vi "Func-Math-Finder-18032016.vi"(4 "All Fn-Math":string[](array[string]), 6 "All Fn Name":string[](array[string]), 7 "Func Name":string, 8 "error in (no error)":errorcluster, 9 "Functions Definition":string[][](table), 11 "Get Tagged String":string) -> (0 "error out":errorcluster, 1 "is empty?":string, 2 "Expression":string)   [LabVIEW 2014]
doc: "This VI takes tagged string from SBML parser.vi as input and translate it into kinetic law. It supports the following five mathematical functions:\n+, -, *, /, pow\n\nDesigned by HB\nhaba@dtu.dk"
uses:
  <vilib>/regexp/Match Regular Expression.xnode
panel:
  out "Fn Variables":string[](array[string])
  out "Nest Fn?":string
  out "Current Args":string[](array[string])
  out "RHS ex":string
  out "Inter. exp":string
  in  "RHS":string
  in  "LHS":string
  # "multiplySOP1k1, addSOP2S1, S2EOP2, subSOP2k1, 4EOP2EOP1"
  # "SOP1 + x 2 EOP1"
  # "SOP1 + SOP2 * a b EOP2 c EOP1"
  # "SOP1 + c SOP2 * a b EOP2 EOP1"
  # "SOP1 + SOP2 * a SOP3 pow x 2 EOP3 EOP2 SOP2 * b x EOP2 c EOP1"
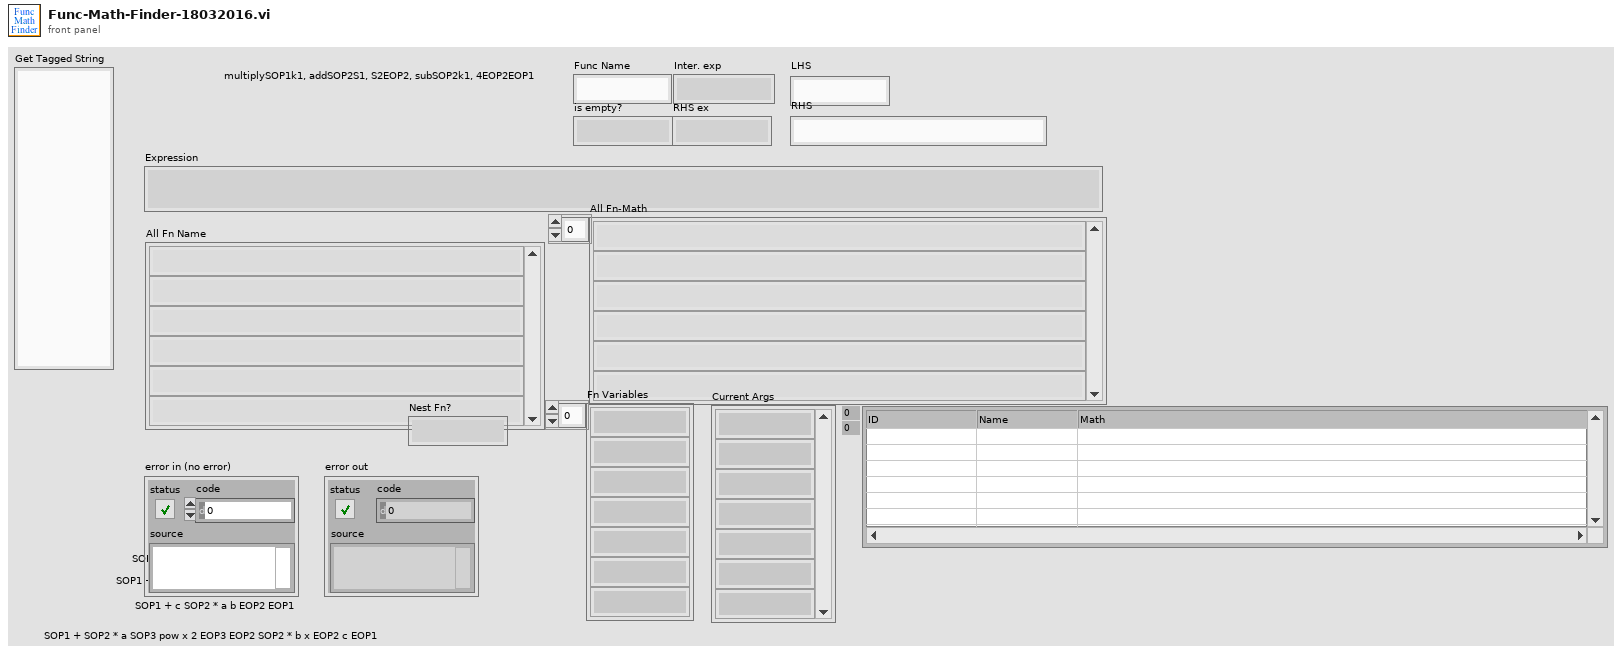
[diagram p1: front panel]
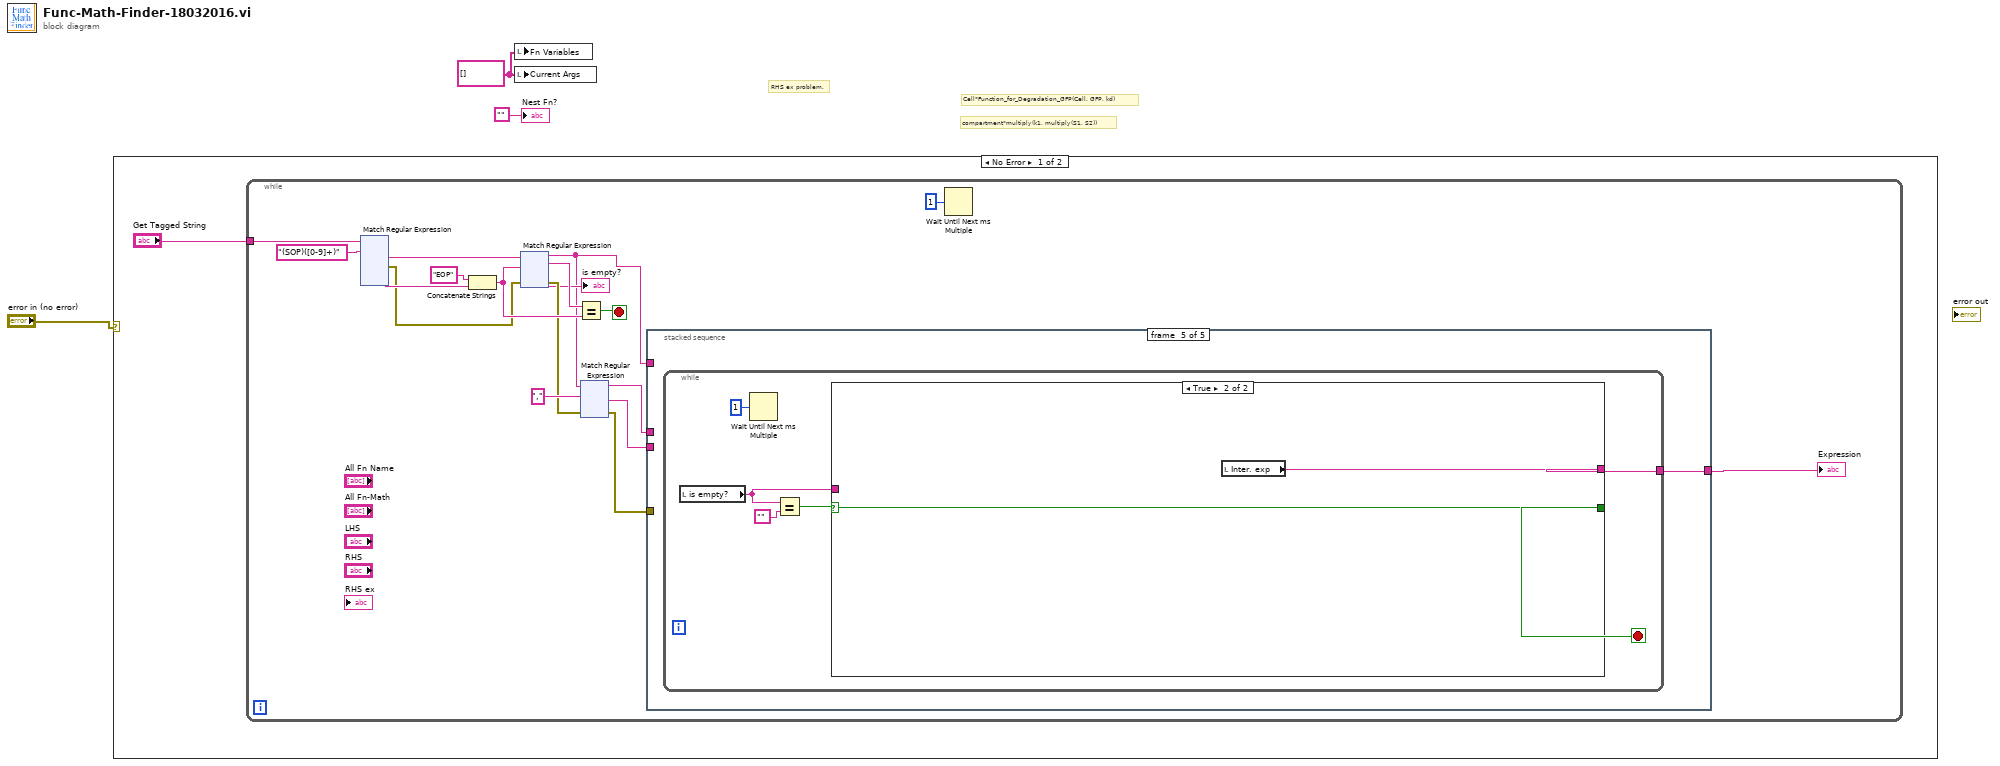
[diagram p0: block diagram]
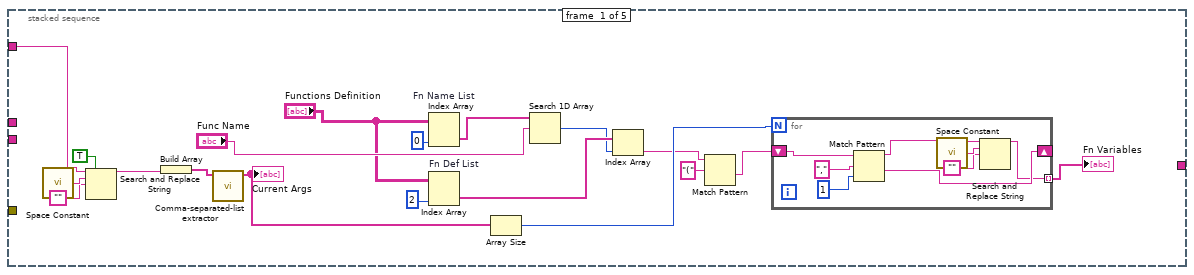
[diagram p2: hidden frame]
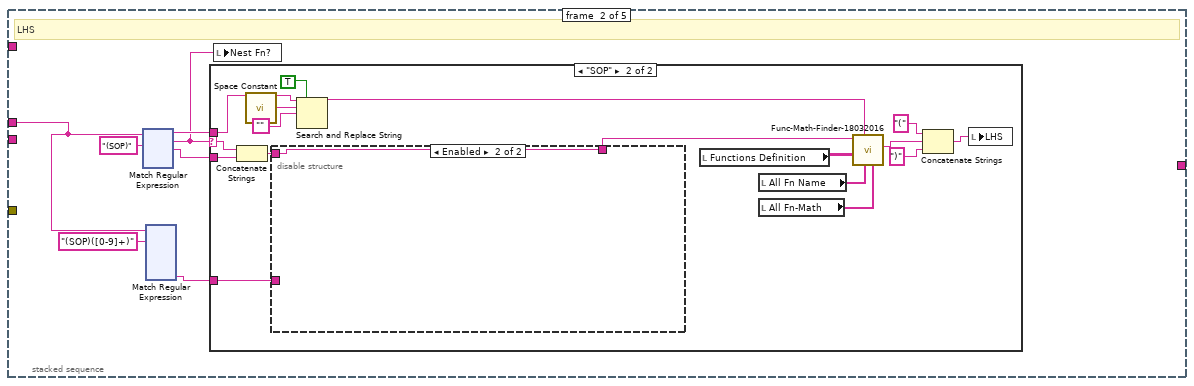
[diagram p3: hidden frame]
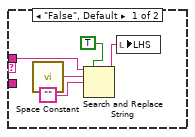
[diagram p4: hidden frame]
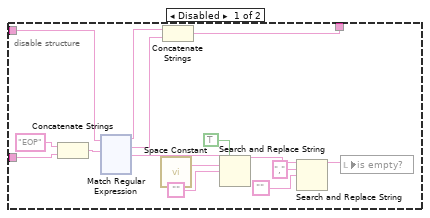
[diagram p5: hidden frame]
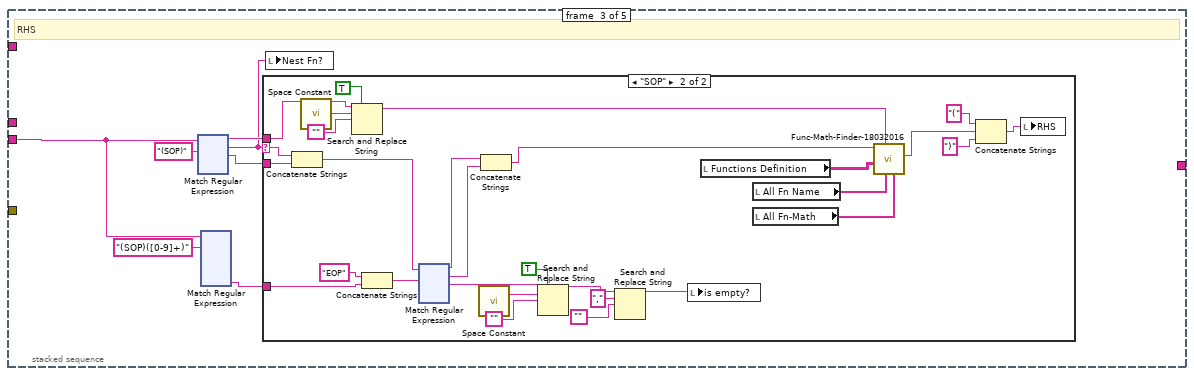
[diagram p6: hidden frame]
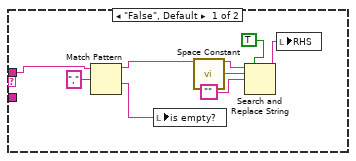
[diagram p7: hidden frame]
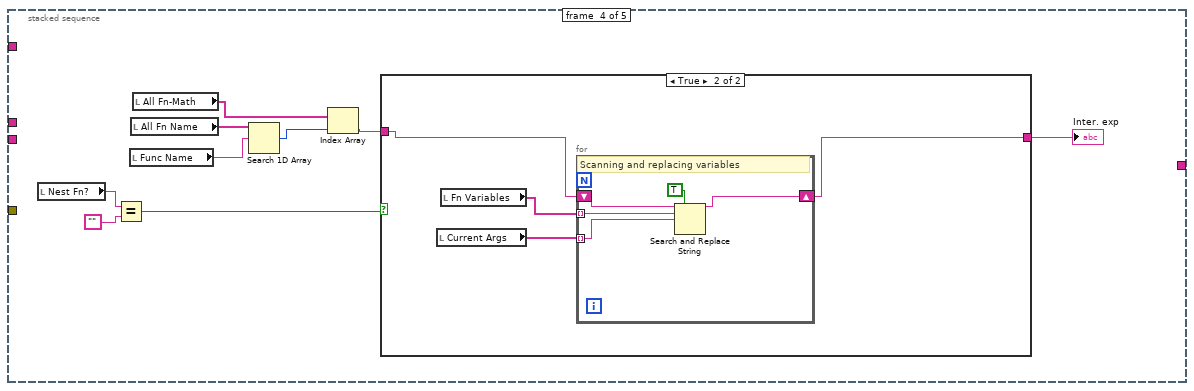
[diagram p8: hidden frame]
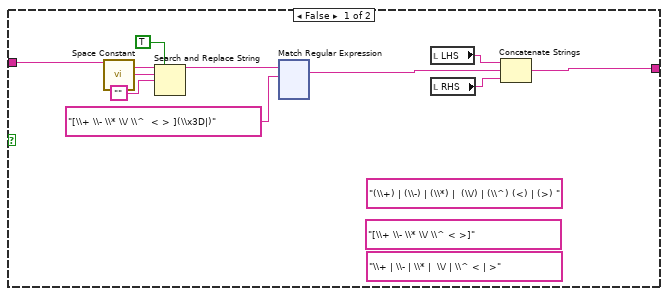
[diagram p9: hidden frame]
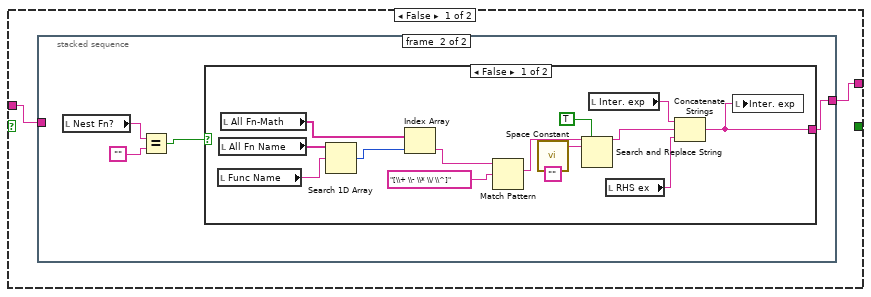
[diagram p10: hidden frame]
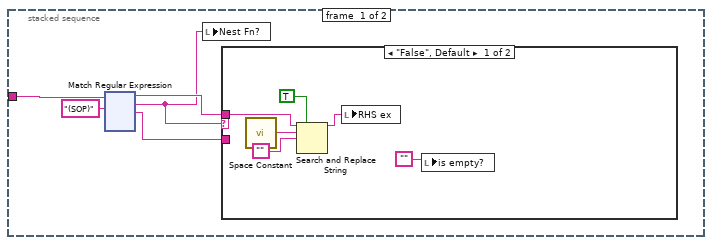
[diagram p11: hidden frame]
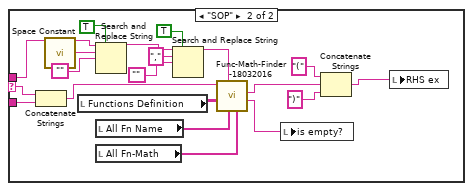
[diagram p12: hidden frame]
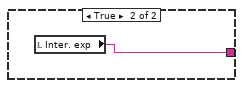
[diagram p13: hidden frame]
diagram:
  w1 = string[] [] ("Current Args")
  # "compartment*multiply(k1, multiply(S1, S2))"
  # "Cell*Function_for_Degradation_GFP(Cell, GFP, kd)"
  # "RHS ex problem."
  n1 = case shown="No Error" "error in (no error)" {
    frame No Error {
      n2 = while {
        tunnel: "Get Tagged String" -> [w14]
        stop <- w20 stop-if-true
        n3 = xnode "Match Regular Expression"("input string"=w14, "regular expression"="(SOP)([0-9]+)") -> ("after match"=w17:string, "error out"=w13:errorcluster, "submatch 2"=w16:string)  [unwired: 4 in, 4 out]
        n4 = Concatenate Strings("EOP" ("regular expression"), w16) -> (w21:string)
        n5 = xnode "Match Regular Expression"("input string"=w17, "regular expression"=w21, "error in"=w13) -> ("before match"=w6:string, "whole match"=w19:string, "after match"=→"is empty?":string, "error out"=w12:errorcluster)  [unwired: 3 in, 1 out]
        n6 = Equal?(x=w19, y=w21) -> (x = y?=w20:bool)
        n7 = xnode "Match Regular Expression"("input string"=w6, "regular expression"="," ("Oprts Lst"), "error in"=w12) -> ("before match"=w11:string, "after match"=w9:string, "error out"=w10:errorcluster)  [unwired: 3 in, 2 out]
        n8 = stacked-sequence {
          tunnel: w11 -> [_ w51 _ _ _]
          tunnel: w10 -> [_ _ _ _ _]
          tunnel: w9 -> [_ _ w442 _ _]
          tunnel: [_ _ _ _ w971] -> w8
          tunnel: w6 -> [w23 _ _ _ _]
          frame #0 {
            n9 = call <vilib>:"Space Constant.vi"() -> ("String"=w26:string)
            n10 = Search and Replace String(replace all?=TRUE ("replace all? (F)"), input string=w23, search string=w26, replace string="") -> (result string=w28:string)  [unwired: 4 in, 3 out]
            n11 = Build Array(w28) -> (w24:string[])
            n12 = call "Comma-separated-list extractor.vi"("In_list"=w24) -> ("List_Out"=w39:string[])  [unwired: 6 in, 1 out]
            "Current Args" <- w39
            n13 = Index Array "Fn Name List"(array="Functions Definition", index (col)=0 ("disabled index (col)")) -> (element=w29:string[])  [unwired: 1 in]
            n14 = Index Array "Fn Def List"(array="Functions Definition", index (col)=2 ("disabled index (col)")) -> (element=w34:string[])  [unwired: 1 in]
            n15 = Array Size(array=w39) -> (size(s)=w40:i32)
            n16 = Search 1D Array(1D array=w29, element="Func Name") -> (index of element=w33:i32)  [unwired: 1 in]
            n17 = Index Array(array=w34, index=w33) -> (element=w38:string)
            n18 = Match Pattern(string=w38, regular expression="(") -> (after substring=w36:string)  [unwired: 1 in, 3 out]
            n19 = for {
              N: w40 -> [_]
              shift-right: [w46] -> _
              shift-left: w36 -> [w49]
              tunnel: [w42] -> w35 mode=indexing
              n20 = Match Pattern(string=w49, regular expression="," ("search string/char (-)"), offset (0)=1) -> (before substring=w43:string, after substring=w46:string)  [unwired: 2 out]
              n21 = call <vilib>:"Space Constant.vi"() -> ("String"=w45:string)
              n22 = Search and Replace String(input string=w43, search string=w45, replace string="") -> (result string=w42:string)  [unwired: 5 in, 3 out]
            }
            "Fn Variables" <- w35
          }
          frame #1 {
            # "LHS"
            n23 = xnode "Match Regular Expression"("input string"=w51, "regular expression"="(SOP)") -> ("before match"=w54:string, "whole match"=w50:string, "after match"=w55:string)  [unwired: 4 in, 2 out]
            n24 = xnode "Match Regular Expression"("input string"=w51, "regular expression"="(SOP)([0-9]+)") -> ("submatch 2"=w52:string)  [unwired: 4 in, 6 out]
            n25 = case shown="\"SOP\"" w50 {
              selector: w50 -> [_ w195]
              tunnel: w54 -> [w175 w186]
              tunnel: w55 -> [_ w194]
              tunnel: w52 -> [_ w182]
              frame "False", Default {
                n26 = call <vilib>:"Space Constant.vi"() -> ("String"=w177:string)
                n27 = Search and Replace String(replace all?=TRUE ("replace all? (F)"), input string=w175, search string=w177, replace string="" ("string")) -> (result string=w174:string)  [unwired: 4 in, 3 out]
                n28 = local write "LHS"(w174) -> ()
              }
              frame "SOP" {
                n29 = Concatenate Strings(w195, w194) -> (w181:string)
                n30 = call <vilib>:"Space Constant.vi"() -> ("String"=w187:string)
                n31 = disable-structure shown="Enabled" {
                  disable-tunnel: w182 -> [w209 _]
                  disable-tunnel: w181 -> [w199 w325]
                  disable-tunnel: [w198 w325] -> w180
                  frame Disabled {
                    n32 = Concatenate Strings("EOP" ("regular expression"), w209) -> (w208:string)
                    n33 = xnode "Match Regular Expression"("input string"=w199, "regular expression"=w208) -> ("before match"=w200:string, "whole match"=w201:string, "after match"=w203:string)  [unwired: 4 in, 2 out]
                    n34 = call <vilib>:"Space Constant.vi"() -> ("String"=w206:string)
                    n35 = Concatenate Strings(w200, w201) -> (w198:string)
                    n36 = Search and Replace String(replace all?=TRUE ("replace all? (F)"), input string=w203, search string=w206, replace string="" ("string")) -> (result string=w205:string)  [unwired: 4 in, 3 out]
                    n37 = Search and Replace String(input string=w205, search string=",", replace string="" ("string")) -> (result string=w202:string)  [unwired: 5 in, 3 out]
                    n38 = local write "is empty?"(w202) -> ()
                  }
                  frame Enabled {
                  }
                }
                n39 = Search and Replace String(replace all?=TRUE ("replace all? (F)"), input string=w186, search string=w187, replace string="" ("string")) -> (result string=w185:string)  [unwired: 4 in, 3 out]
                n40 = local read "Functions Definition"() -> (w179:string[][])
                n41 = local read "All Fn Name"() -> (w184:string[])
                n42 = local read "All Fn-Math"() -> (w183:string[])
                n43 = call "Func-Math-Finder-18032016.vi"("All Fn-Math"=w183, "All Fn Name"=w184, "Func Name"=w185, "Functions Definition"=w179, "Get Tagged String"=w180) -> ("Expression"=w190:string)  [unwired: 4 in, 2 out]
                n44 = Concatenate Strings("(" ("string"), w190, ")" ("string")) -> (w191:string)
                n45 = local write "LHS"(w191) -> ()
              }
            }
            n46 = local write "Nest Fn?"(w50) -> ()
          }
          frame #2 {
            # "RHS"
            n47 = xnode "Match Regular Expression"("input string"=w442, "regular expression"="(SOP)") -> ("before match"=w444:string, "whole match"=w440:string, "after match"=w445:string)  [unwired: 4 in, 2 out]
            n48 = xnode "Match Regular Expression"("input string"=w442, "regular expression"="(SOP)([0-9]+)") -> ("submatch 2"=w441:string)  [unwired: 4 in, 6 out]
            n49 = case shown="\"SOP\"" w440 {
              selector: w440 -> [_ w600]
              tunnel: w444 -> [w567 w591]
              tunnel: w445 -> [_ w599]
              tunnel: w441 -> [_ w586]
              frame "False", Default {
                n50 = Match Pattern(string=w567, regular expression=",") -> (before substring=w565:string, after substring=w564:string)  [unwired: 1 in, 2 out]
                n51 = local write "is empty?"(w564) -> ()
                n52 = call <vilib>:"Space Constant.vi"() -> ("String"=w570:string)
                n53 = Search and Replace String(replace all?=TRUE ("replace all? (F)"), input string=w565, search string=w570, replace string="" ("string")) -> (result string=w568:string)  [unwired: 4 in, 3 out]
                n54 = local write "RHS"(w568) -> ()
              }
              frame "SOP" {
                n55 = Concatenate Strings(w600, w599) -> (w576:string)
                n56 = call <vilib>:"Space Constant.vi"() -> ("String"=w592:string)
                n57 = Search and Replace String(replace all?=TRUE ("replace all? (F)"), input string=w591, search string=w592, replace string="" ("string")) -> (result string=w590:string)  [unwired: 4 in, 3 out]
                n58 = Concatenate Strings("EOP" ("regular expression"), w586) -> (w585:string)
                n59 = xnode "Match Regular Expression"("input string"=w576, "regular expression"=w585) -> ("before match"=w577:string, "whole match"=w578:string, "after match"=w580:string)  [unwired: 4 in, 2 out]
                n60 = call <vilib>:"Space Constant.vi"() -> ("String"=w583:string)
                n61 = Concatenate Strings(w577, w578) -> (w575:string)
                n62 = Search and Replace String(replace all?=TRUE ("replace all? (F)"), input string=w580, search string=w583, replace string="" ("string")) -> (result string=w582:string)  [unwired: 4 in, 3 out]
                n63 = Search and Replace String(input string=w582, search string=",", replace string="" ("string")) -> (result string=w579:string)  [unwired: 5 in, 3 out]
                n64 = local write "is empty?"(w579) -> ()
                n65 = local read "Functions Definition"() -> (w572:string[][])
                n66 = local read "All Fn Name"() -> (w589:string[])
                n67 = local read "All Fn-Math"() -> (w588:string[])
                n68 = call "Func-Math-Finder-18032016.vi"("All Fn-Math"=w588, "All Fn Name"=w589, "Func Name"=w590, "Functions Definition"=w572, "Get Tagged String"=w575) -> ("Expression"=w595:string)  [unwired: 4 in, 2 out]
                n69 = Concatenate Strings("(" ("string"), w595, ")" ("string")) -> (w596:string)
                n70 = local write "RHS"(w596) -> ()
              }
            }
            n71 = local write "Nest Fn?"(w440) -> ()
          }
          frame #3 {
            n72 = local read "Nest Fn?"() -> (w836:string)
            n73 = Equal?(x=w836, y="") -> (x = y?=w837:bool)
            n74 = local read "Func Name"() -> (w830:string)
            n75 = local read "All Fn Name"() -> (w832:string[])
            n76 = local read "All Fn-Math"() -> (w831:string[])
            n77 = Search 1D Array(1D array=w832, element=w830) -> (index of element=w833:i32)  [unwired: 1 in]
            n78 = Index Array(array=w831, index=w833) -> (element=w829:string)
            n79 = case shown="True" w837 {
              tunnel: [w839 w962] -> w834
              tunnel: w829 -> [w838 w963]
              frame False {
                (unwired) "[\\+ \\- \\* \\/ \\^ < >]" ("Oprts Lst")
                (unwired) "\\+ | \\- | \\* |  \\/ | \\^ < | >" ("Oprts Lst")
                (unwired) "(\\+) | (\\-) | (\\*) |  (\\/) | (\\^) (<) | (>) " ("Oprts Lst")
                n80 = call <vilib>:"Space Constant.vi"() -> ("String"=w843:string)
                n81 = Search and Replace String(replace all?=TRUE ("replace all? (F)"), input string=w838, search string=w843, replace string="" ("string")) -> (result string=w840:string)  [unwired: 4 in, 3 out]
                n82 = xnode "Match Regular Expression"("input string"=w840, "regular expression"="[\\+ \\- \\* \\/ \\^  < > ](\\x3D|)" ("Oprts Lst")) -> ("whole match"=w841:string)  [unwired: 4 in, 4 out]
                n83 = local read "LHS"() -> (w847:string)
                n84 = local read "RHS"() -> (w846:string)
                n85 = Concatenate Strings(w847, w841, w846) -> (w839:string)
              }
              frame True {
                n86 = local read "Current Args"() -> (w964:string[])
                n87 = local read "Fn Variables"() -> (w965:string[])
                n88 = for {
                  tunnel: w965 -> [w969] mode=indexing
                  tunnel: w964 -> [w968] mode=indexing
                  shift-right: [w966] -> w962
                  shift-left: w963 -> [w970]
                  # "Scanning and replacing variables"
                  n89 = Search and Replace String(replace all?=TRUE ("replace all? (F)"), input string=w970, search string=w969, replace string=w968) -> (result string=w966:string)  [unwired: 4 in, 3 out]
                }
              }
            }
            "Inter. exp" <- w834
          }
          frame #4 {
            n90 = while {
              tunnel: [w974] -> w971
              stop <- w975 stop-if-true
              n91 = local read "is empty?"() -> (w973:string)
              n92 = Wait Until Next ms Multiple(millisecond multiple=u32 1 ("milliseconds to wait")) -> ()  [unwired: 1 out]
              n93 = Equal?(x=w973, y="") -> (x = y?=w976:bool)
              n94 = case shown="True" w976 {
                selector: w976 -> [_ w1144]
                tunnel: [_ w1144] -> w975
                tunnel: [w978 w1143] -> w974
                tunnel: w973 -> [w979 _]
                frame False {
                  n95 = stacked-sequence {
                    tunnel: w979 -> [w981 _]
                    tunnel: [_ w1128] -> w978
                    frame #0 {
                      n96 = xnode "Match Regular Expression"("input string"=w981, "regular expression"="(SOP)") -> ("before match"=w982:string, "whole match"=w980:string, "after match"=w983:string)  [unwired: 4 in, 2 out]
                      n97 = local write "Nest Fn?"(w980) -> ()
                      n98 = case shown="\"False\", Default" w980 {
                        selector: w980 -> [_ w1010]
                        tunnel: w982 -> [w987 w1000]
                        tunnel: w983 -> [_ w1009]
                        frame "False", Default {
                          n99 = call <vilib>:"Space Constant.vi"() -> ("String"=w989:string)
                          n100 = Search and Replace String(replace all?=TRUE ("replace all? (F)"), input string=w987, search string=w989, replace string="" ("string")) -> (result string=w986:string)  [unwired: 4 in, 3 out]
                          n101 = local write "RHS ex"(w986) -> ()
                          n102 = local write "is empty?"("") -> ()
                        }
                        frame "SOP" {
                          n103 = Concatenate Strings(w1010, w1009) -> (w1008:string)
                          n104 = call <vilib>:"Space Constant.vi"() -> ("String"=w1001:string)
                          n105 = local read "Functions Definition"() -> (w991:string[][])
                          n106 = Search and Replace String(replace all?=TRUE ("replace all? (F)"), input string=w1000, search string=w1001, replace string="" ("string")) -> (result string=w995:string)  [unwired: 4 in, 3 out]
                          n107 = local read "All Fn Name"() -> (w999:string[])
                          n108 = local read "All Fn-Math"() -> (w998:string[])
                          n109 = Search and Replace String(replace all?=TRUE ("replace all? (F)"), input string=w995, search string=",", replace string="" ("string")) -> (result string=w993:string)  [unwired: 4 in, 3 out]
                          n110 = call "Func-Math-Finder-18032016.vi"("All Fn-Math"=w998, "All Fn Name"=w999, "Func Name"=w993, "Functions Definition"=w991, "Get Tagged String"=w1008) -> ("is empty?"=w992:string, "Expression"=w1004:string)  [unwired: 4 in, 1 out]
                          n111 = local write "is empty?"(w992) -> ()
                          n112 = Concatenate Strings("(" ("string"), w1004, ")" ("string")) -> (w1005:string)
                          n113 = local write "RHS ex"(w1005) -> ()
                        }
                      }
                    }
                    frame #1 {
                      n114 = local read "Nest Fn?"() -> (w1127:string)
                      n115 = Equal?(x=w1127, y="") -> (x = y?=w1125:bool)
                      n116 = case shown="False" w1125 {
                        tunnel: [w1136 w1142] -> w1128
                        frame False {
                          (unwired) "" ("string")
                          n117 = local read "Func Name"() -> (w1130:string)
                          n118 = local read "All Fn Name"() -> (w1132:string[])
                          n119 = local read "All Fn-Math"() -> (w1131:string[])
                          n120 = Search 1D Array(1D array=w1132, element=w1130) -> (index of element=w1134:i32)  [unwired: 1 in]
                          n121 = Index Array(array=w1131, index=w1134) -> (element=w1133:string)
                          n122 = Match Pattern(string=w1133, regular expression="[\\+ \\- \\* \\/ \\^]" ("Oprts Lst")) -> (match substring=w1129:string)  [unwired: 1 in, 3 out]
                          n123 = call <vilib>:"Space Constant.vi"() -> ("String"=w1140:string)
                          n124 = Search and Replace String(replace all?=TRUE ("replace all? (F)"), input string=w1129, search string=w1140) -> (result string=w1139:string)  [unwired: 5 in, 3 out]
                          n125 = local read "Inter. exp"() -> (w1138:string)
                          n126 = local read "RHS ex"() -> (w1137:string)
                          n127 = Concatenate Strings(w1138, w1139, w1137) -> (w1136:string)
                          n128 = local write "Inter. exp"(w1136) -> ()
                        }
                        frame True {
                          n129 = local read "Inter. exp"() -> (w1142:string)
                        }
                      }
                    }
                  }
                }
                frame True {
                  n130 = local read "Inter. exp"() -> (w1143:string)
                }
              }
            }
          }
        }
        "Expression" <- w8
        n131 = Wait Until Next ms Multiple(millisecond multiple=u32 1 ("milliseconds to wait")) -> ()  [unwired: 1 out]
      }
    }
    frame Error {
    }
  }
  n132 = local write "Fn Variables"(w1) -> ()
  n133 = local write "Current Args"(w1) -> ()
  "Nest Fn?" <- ""
